vi "ex_3.vi"() -> ()   [LabVIEW 2020]
panel:
  in  "stop":bool
  out "Time Elapsed?":bool
  in  "Time Limit":dbl
  in  "Reset (T)/Count (F)":bool
  out "Numeric":dbl format="%#.2f"
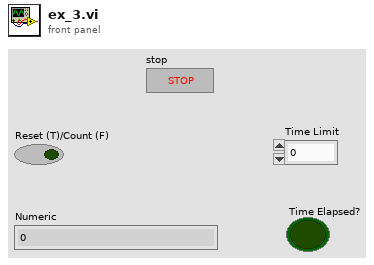
[diagram p1: front panel]
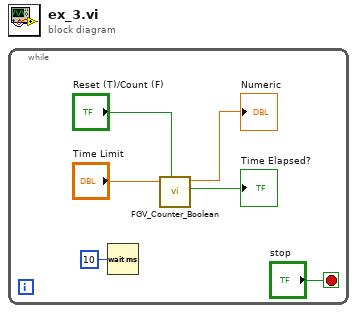
[diagram p0: block diagram]
diagram:
  n1 = while {
    stop <- "stop" stop-if-true
    n2 = Wait (ms)(milliseconds to wait=u32 10) -> ()  [unwired: 1 out]
    n3 = call "FGV_Counter_Boolean.vi"("Reset (T)/Count (F)"="Reset (T)/Count (F)", "Time Limit (10)"="Time Limit") -> ("Time Elapsed?"=→"Time Elapsed?":bool, "Time"=→"Numeric":dbl)  [unwired: 7 in, 1 out]
  }
